vi "sv_UFF58GetChannelLength.vi"(0 "channel refnum":refnum<k20>, 11 "error in":errorcluster caption="error in (no error)") -> (4 "dup channel refnum":refnum<k20>, 6 "channel length":i32, 15 "error out":errorcluster)   [LabVIEW 2017, in "SoundVib_UFF58.lvlib"]
doc: "This VI returns the <B>channel length</B> for the given <B>channel refnum</B>"
uses:
  <vilib>/addons/Sound and Vibration/svt_UFF58/SoundVib_UFF58.lvlib
  <vilib>/Platform/storage/Storage.llb/Get Property (I32).vi
  <vilib>/Platform/storage/Storage.llb/Get Property (Storage Refnum).vi
  <vilib>/Platform/storage/Storage.llb/Get Property (Storage Refnums).vi
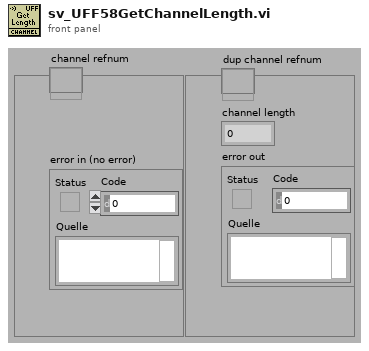
[diagram p1: front panel]
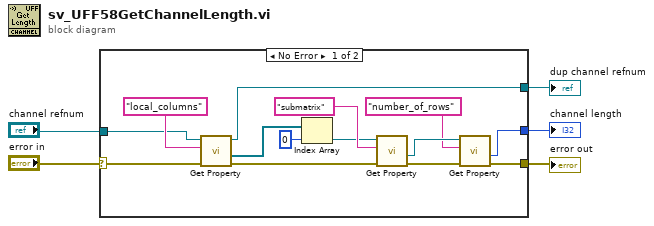
[diagram p0: block diagram]
diagram:
  n1 = case shown="No Error" "error in" {
    selector: "error in" -> [w6 w21]
    tunnel: [w19 _] -> w5
    tunnel: [w17 w21] -> w4
    tunnel: "channel refnum" -> [w8 w20]
    tunnel: [w7 w20] -> w2
    frame No Error {
      n2 = call-poly <vilib>:"Get Property.vi"("error in (no error)"=w6, "Property name"="local_columns" ("property name"), "storage refnum"=w8) -> ("error out"=w15:errorcluster, "Value"=w10:refnum<k20>[], "storage refnum out"=w7:refnum<k20>)  [unwired: 6 in]
      n3 = Index Array(array=w10, index=0 ("Index")) -> (element=w12:refnum<k20>)
      n4 = call-poly <vilib>:"Get Property.vi"("error in (no error)"=w15, "Property name"="submatrix" ("property name"), "storage refnum"=w12) -> ("error out"=w16:errorcluster, "Value"=w18:refnum<k20>)  [unwired: 6 in, 1 out]
      n5 = call-poly <vilib>:"Get Property.vi"("error in (no error)"=w16, "Property name"="number_of_rows" ("property name"), "storage refnum"=w18) -> ("error out"=w17:errorcluster, "Value"=w19:i32)  [unwired: 6 in, 1 out]
    }
    frame Error {
    }
  }
  "channel length" <- w5
  "error out" <- w4
  "dup channel refnum" <- w2
